vi "Test_ReadValue_TransportClosed_ReadError.vi"(8 "error in (no error)":errorcluster, 11 "TestCase in":refnum<class "TestQueueTransport.lvclass">) -> (0 "error out":errorcluster, 3 "TestCase out":refnum<class "TestQueueTransport.lvclass">)   [LabVIEW 2017, in "TestQueueTransport.lvclass"]
uses:
  TestQueueTransport.lvclass
  Source/Concrete/QueueTransport/QueueTransport.lvclass/QueueTransport.ctl
  <vilib>/Utility/error.llb/Error Cluster From Error Code.vi
  Source/Concrete/QueueTransport/QueueTransport.lvclass
panel:
  out "Return Error":errorcluster
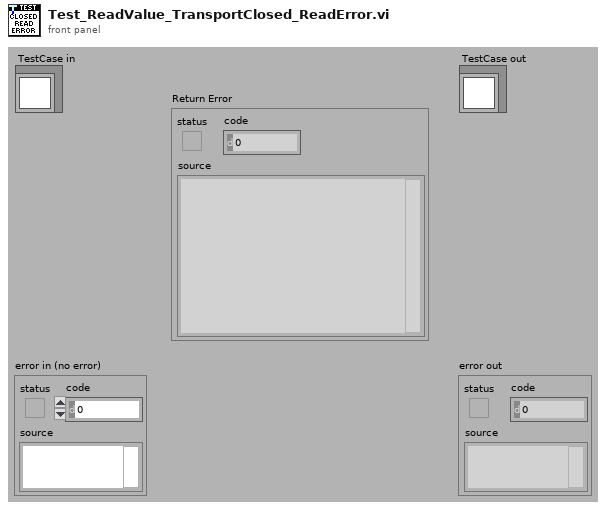
[diagram p1: front panel]
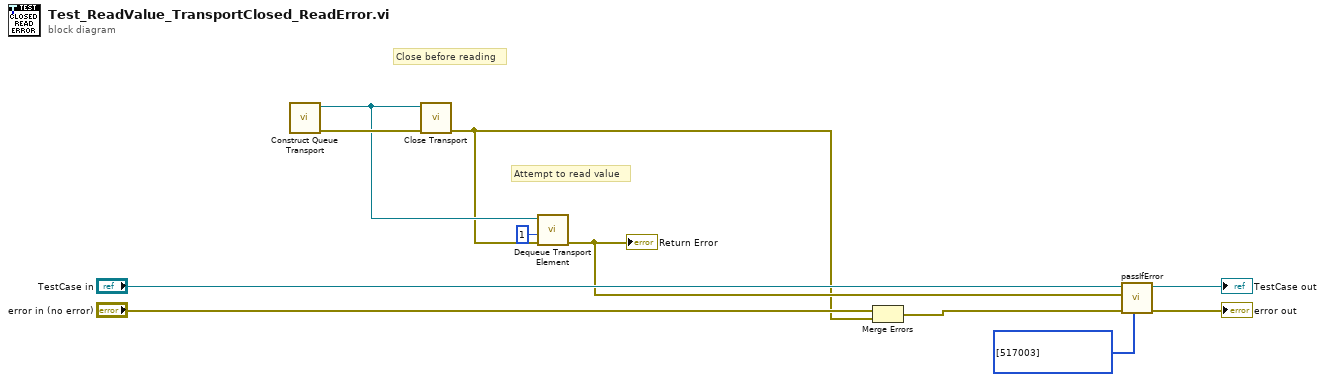
[diagram p0: block diagram]
diagram:
  # "Close before reading"
  # "Attempt to read value"
  n1 = call "Construct Queue Transport.vi"() -> ("error out"=w4:errorcluster, "QueueTransport"=w3:refnum<class "QueueTransport.lvclass">)  [unwired: 10 in]
  n2 = call-dynamic "Close Transport.vi"("error in (no error)"=w4, "QueueTransport"=w3) -> ("error out"=w1:errorcluster)  [unwired: 9 in]
  n3 = call "Dequeue Transport Element.vi"("error in (no error)"=w1, "Timeout In ms (-1)"=1, "QueueTransport"=w3) -> ("error out"=w2:errorcluster)  [unwired: 5 in, 3 out]
  "Return Error" <- w2
  n4 = Merge Errors("error in (no error)", w1) -> (w6:errorcluster)
  n5 = call-dynamic "passIfError.vi"("passing error codes (default = any error code)"=i32[] [517003], "error in (no error)"=w6, "error"=w2, "TestCase in"="TestCase in") -> ("error out"=→"error out":errorcluster, "TestCase out"=→"TestCase out":refnum<class "TestQueueTransport.lvclass">)  [unwired: 6 in]
